vi "Status.vi"(7 "Action":T2(ring), 8 "error in":errorcluster, 10 "Diglett":refnum<vi>, 11 "semaphore":T1) -> (0 "error out":errorcluster, 3 "semaphore":T1)   [LabVIEW 2011]
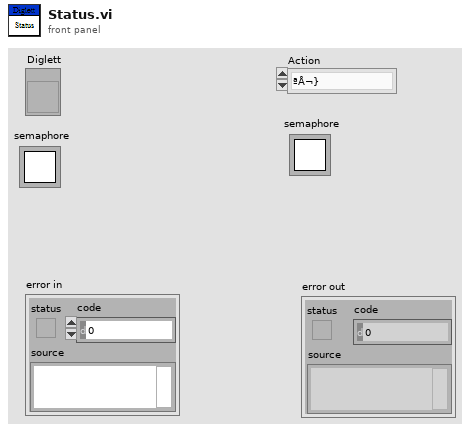
[diagram p1: front panel]
types:
  T1 = typedef "Semaphore RefNum" = refnum<k1>
  T2 = enum16{"ªÅ¬}", "¦a¹«¤É°_", "¦a¹«¤U­°", "¦a¹«³Q¥´", "¥´¿ù¬}"}
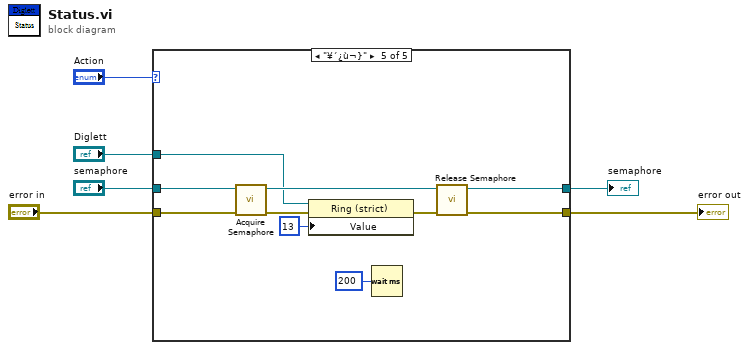
[diagram p0: block diagram]
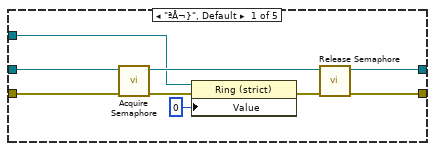
[diagram p2: hidden frame]
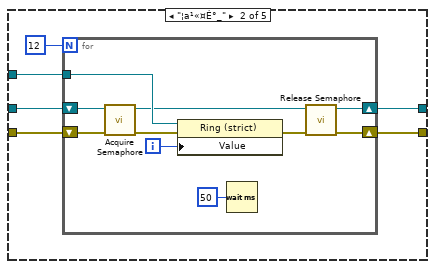
[diagram p3: hidden frame]
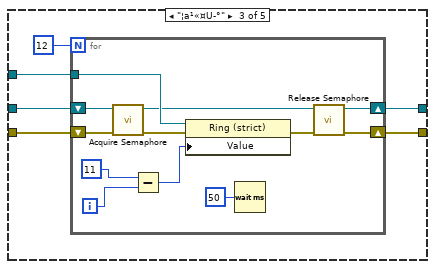
[diagram p4: hidden frame]
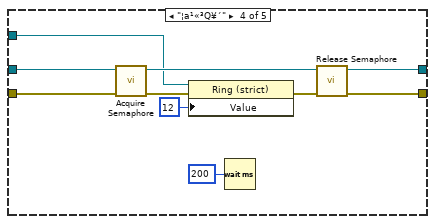
[diagram p5: hidden frame]
diagram:
  n1 = case shown="\"¥´¿ù¬}\"" "Action" {
    tunnel: "Diglett" -> [w10 w20 w34 w54 w64]
    tunnel: "error in" -> [w12 w19 w36 w56 w66]
    tunnel: [w9 w18 w35 w53 w63] -> w3
    tunnel: "semaphore" -> [w11 w17 w33 w55 w65]
    tunnel: [w7 w16 w32 w50 w60] -> w1
    frame "ªÅ¬}", Default {
      n2 = call <vilib>:"Acquire Semaphore.vi"("error in (no error)"=w12, "semaphore"=w11) -> ("error out"=w13:errorcluster, "semaphore out"=w15:T1)  [unwired: 3 in, 1 out]
      n3 = property class="Ring (strict)"(reference=w10, error in=w13, "Value"=u16 0) -> (error out=w14:errorcluster)  [unwired: 1 out]
      n4 = call <vilib>:"Release Semaphore.vi"("error in (no error)"=w14, "semaphore"=w15) -> ("error out"=w9:errorcluster, "semaphore out"=w7:T1)  [unwired: 4 in]
    }
    frame "¦a¹«¤É°_" {
      n5 = for {
        N: 12 -> [_]
        tunnel: w20 -> [w31]
        shift-right: [w25] -> w18
        shift-left: w19 -> [w27]
        shift-right: [w22] -> w16
        shift-left: w17 -> [w23]
        i -> [w30]
        n6 = call <vilib>:"Acquire Semaphore.vi"("error in (no error)"=w27, "semaphore"=w23) -> ("error out"=w28:errorcluster, "semaphore out"=w24:T1)  [unwired: 3 in, 1 out]
        n7 = property class="Ring (strict)"(reference=w31, error in=w28, "Value"=w30) -> (error out=w26:errorcluster)  [unwired: 1 out]
        n8 = Wait (ms)(milliseconds to wait=u32 50) -> ()  [unwired: 1 out]
        n9 = call <vilib>:"Release Semaphore.vi"("error in (no error)"=w26, "semaphore"=w24) -> ("error out"=w25:errorcluster, "semaphore out"=w22:T1)  [unwired: 4 in]
      }
    }
    frame "¦a¹«¤U­°" {
      n10 = for {
        N: 12 -> [_]
        tunnel: w34 -> [w49]
        shift-right: [w44] -> w35
        shift-left: w36 -> [w46]
        shift-right: [w38] -> w32
        shift-left: w33 -> [w42]
        i -> [w41]
        n11 = call <vilib>:"Acquire Semaphore.vi"("error in (no error)"=w46, "semaphore"=w42) -> ("error out"=w47:errorcluster, "semaphore out"=w43:T1)  [unwired: 3 in, 1 out]
        n12 = Subtract(x=11, y=w41) -> (x-y=w39:i32)
        n13 = property class="Ring (strict)"(reference=w49, error in=w47, "Value"=w39) -> (error out=w45:errorcluster)  [unwired: 1 out]
        n14 = Wait (ms)(milliseconds to wait=u32 50) -> ()  [unwired: 1 out]
        n15 = call <vilib>:"Release Semaphore.vi"("error in (no error)"=w45, "semaphore"=w43) -> ("error out"=w44:errorcluster, "semaphore out"=w38:T1)  [unwired: 4 in]
      }
    }
    frame "¦a¹«³Q¥´" {
      n16 = call <vilib>:"Acquire Semaphore.vi"("error in (no error)"=w56, "semaphore"=w55) -> ("error out"=w57:errorcluster, "semaphore out"=w59:T1)  [unwired: 3 in, 1 out]
      n17 = property class="Ring (strict)"(reference=w54, error in=w57, "Value"=u16 12) -> (error out=w58:errorcluster)  [unwired: 1 out]
      n18 = Wait (ms)(milliseconds to wait=u32 200) -> ()  [unwired: 1 out]
      n19 = call <vilib>:"Release Semaphore.vi"("error in (no error)"=w58, "semaphore"=w59) -> ("error out"=w53:errorcluster, "semaphore out"=w50:T1)  [unwired: 4 in]
    }
    frame "¥´¿ù¬}" {
      n20 = call <vilib>:"Acquire Semaphore.vi"("error in (no error)"=w66, "semaphore"=w65) -> ("error out"=w67:errorcluster, "semaphore out"=w69:T1)  [unwired: 3 in, 1 out]
      n21 = property class="Ring (strict)"(reference=w64, error in=w67, "Value"=u16 13) -> (error out=w68:errorcluster)  [unwired: 1 out]
      n22 = Wait (ms)(milliseconds to wait=u32 200) -> ()  [unwired: 1 out]
      n23 = call <vilib>:"Release Semaphore.vi"("error in (no error)"=w68, "semaphore"=w69) -> ("error out"=w63:errorcluster, "semaphore out"=w60:T1)  [unwired: 4 in]
    }
  }
  "error out" <- w3
  "semaphore" <- w1
